vi "PH_PSDBWriter.check PSDB writing condition.vi"(0 "i ref in":refnum<vi>, 2 "wanted Subsystem":T1 caption="PHELIX Subsysteme" items=["Miscellaneous", "fs-Frontend", "ns-Frontend", "PreAmp", "MainAmp", "MAS", "COS", "Beamline", "Experiment Laserbay", "Experiment Laserlabor", "Experiment Z6", "Timing", "Pulsed Power"], 5 "error IO":errorcluster) -> (14 "i ref out":refnum<vi>, 17 "write PSDB?":bool, 19 "error out":errorcluster)   [LabVIEW 2014, in "PH_PSDBWriter.lvlib"]
doc: "This VI checks whether data shall be send to the PSDB: If the wanted subsystem is not -1, equals the own subsystem and if the data status is not \"no data collection, the output is true."
uses:
  PH_PSDBWriter.lvlib
  PH_PSDBWriter.PHELIX-Subsystems.ctl
  PH_PSDBWriter.Data Status.ctl
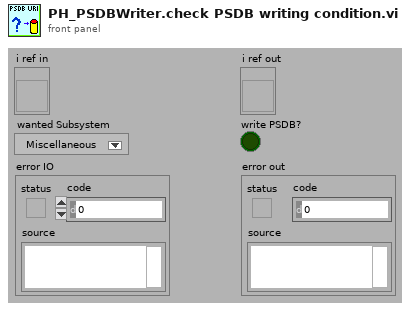
[diagram p1: front panel]
types:
  T1 = typedef "PH_PSDBWriter.lvlib/PH_PSDBWriter.PHELIX-Subsystems.ctl" = i32
  T2 = typedef "PH_PSDBWriter.lvlib/PH_PSDBWriter.Data Status.ctl" = i16
  T3 = typedef "PH_PSDBWriter.lvlib/PH_PSDBWriter.i attribute.ctl" = cluster{"PSDB Status Service ID":i32, "Instance ID":i32, "Shot #":i32, "Subsystem":T1, "Data Status":T2, "Ref PSDB Status":refnum<vi>, "PSDB Error Code":i32, "PSDB Dataset":T4, "PSDB Thread":cluster{"Ref":refnum<vi>, "Q-Ref":refnum<queue>}, "PSDB Credentials":T12}
  T4 = typedef "PH_PSDBWriter.lvlib/PH_PSDBWriter.PSDB Dataset.ctl" = cluster{"Version":i32, "2D data Input":T5[], "Boolean Input":T7[], "Image Input":T8[], "Numeric Input":T10[], "String Input":T11[]}
  T5 = typedef "PH_PSDBWriter.lvlib/PH_PSDBWriter.2D dataset.ctl" = cluster{"name":string, "data":dbl[][], "axis description":T6}
  T6 = typedef "PSDB.lvlib/PSDB_AxisDescription.ctl" = cluster{"x axis label":string, "y axis label":string, "x axis unit":string, "y axis unit":string}
  T7 = typedef "PH_PSDBWriter.lvlib/PH_PSDBWriter.Boolean dataset.ctl" = cluster{"name":string, "data":bool, "unit":string}
  T8 = typedef "PH_PSDBWriter.lvlib/PH_PSDBWriter.Image dataset.ctl" = cluster{"name":string, "data":T9, "unit":string}
  T9 = typedef "IMAQ Image.ctl" = refnum<image>
  T10 = typedef "PH_PSDBWriter.lvlib/PH_PSDBWriter.Numeric dataset.ctl" = cluster{"name":string, "data":dbl, "unit":string}
  T11 = typedef "PH_PSDBWriter.lvlib/PH_PSDBWriter.String dataset.ctl" = cluster{"name":string, "data":string, "unit":string}
  T12 = typedef "PH_Common.lvlib/PH_Connection.PSDB Credentials.ctl" = cluster{"PW":string, "ID":string, "DS":string}
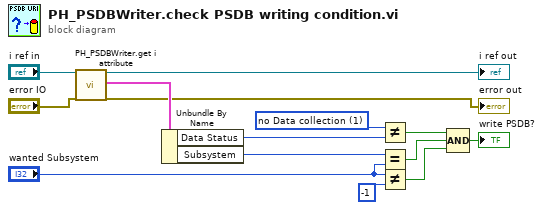
[diagram p0: block diagram]
diagram:
  w8 = T2 1 items=["no info", "no Data collection", "no problem", "Error getting the instance ID", "Error writing Data to data base", "Error concerning the subsystem"] ("Metadata.Data Status")
  n1 = call "PH_PSDBWriter.get i attribute.vi"("i ref in"="i ref in", "error in (no error)"="error IO") -> ("i ref out"=→"i ref out":refnum<vi>, "i attribute"=w12:T3, "error out"=→"error out":errorcluster)  [unwired: 15 in]
  n2 = Unbundle By Name(w12) -> ("Data Status"=w7:T2, "Subsystem"=w11:T1)
  n3 = Not Equal?(x=w8, y=w7) -> (x != y?=w4:bool)
  n4 = Equal?(x=w11, y="wanted Subsystem") -> (x = y?=w3:bool)
  n5 = Not Equal?(x="wanted Subsystem", y=-1) -> (x != y?=w2:bool)
  n6 = Compound Arithmetic op=AND(w4, w3, w2) -> (→"write PSDB?":bool)
